vi "AO Create Channel.vi"(8 "error in (no error)":errorcluster, 10 "Analog Configuration":T1, 11 "C100L in":refnum<class "C100L.lvclass">) -> (0 "error out":errorcluster, 3 "C100L out":refnum<class "C100L.lvclass">)   [LabVIEW 2021, in "C100L.lvlib" / "C100L.lvclass"]
uses:
  C100L.lvclass
  DAQ-arch/Analog Configure.ctl
  C100L.lvclass/C100L.ctl
  DAQ-arch/Analog Output On Demand/Analog Output On Demand/Analog Output On Demand.lvclass
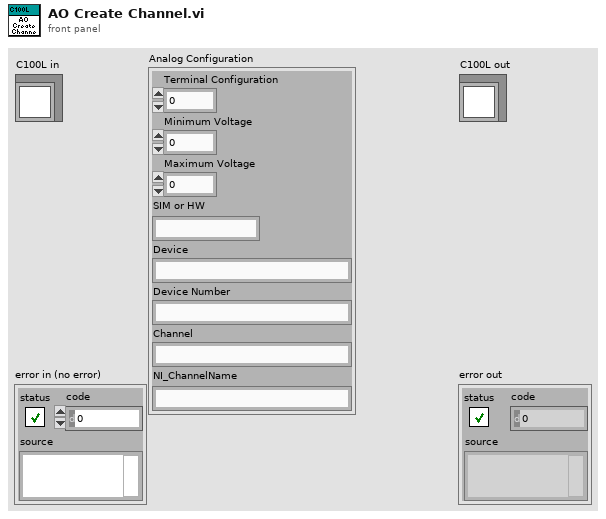
[diagram p1: front panel]
types:
  T1 = typedef "Analog Configure.ctl" = cluster{"Terminal Configuration":i32, "Minimum Voltage":dbl, "Maximum Voltage":dbl, "SIM or HW":string, "Device":string, "Device Number":string, "Channel":string, "NI_ChannelName":string}
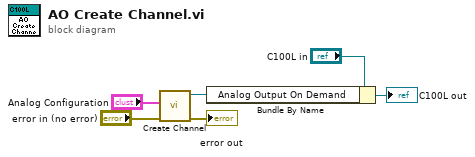
[diagram p0: block diagram]
diagram:
  n1 = call "Create Channel.vi"("error in (no error)"="error in (no error)", "Analog Configuration"="Analog Configuration") -> ("error out"=→"error out":errorcluster, "Analog Output On Demand out"=w4:refnum<class "Analog Output On Demand.lvclass">)  [unwired: 8 in]
  n2 = Bundle By Name(cluster="C100L in", "Analog Output On Demand"=w4) -> (→"C100L out":refnum<class "C100L.lvclass">)
